vi "add set temp(SubVI).vi"(10 "字符串":string) -> (0 "布尔 3":bool, 2 "连接的字符串":string)   [LabVIEW 2019, in "SubVI.lvlib"]
uses:
  SubVI.lvlib
panel:
  in  "Mode":i32(ring) items=["FastSettle", "NoOvershoot"]
  in  "cancel":bool
  in  "ok":bool
  in  "Rate(K/min)":dbl=10.0 min=0.0 max=10.0
  in  "Temperature(K)":dbl=2.0 min=2.0 max=400.0
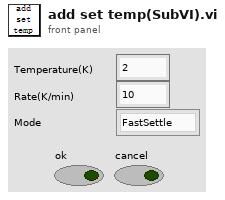
[diagram p1: front panel]
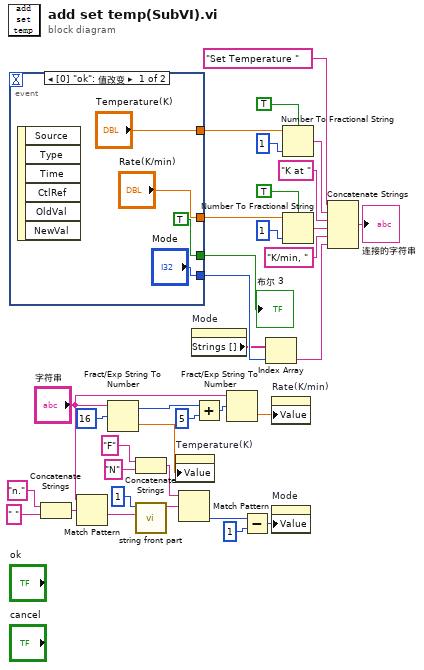
[diagram p0: block diagram]
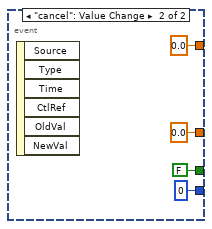
[diagram p2: hidden frame]
diagram:
  n1 = event shown="[0] \"ok\": 值改变" {
    selector: _ -> [_ _]
    dyn-events: _ -> [_ _]
    timeout: _ -> [_ _]
    tunnel: ["Rate(K/min)" 0.0 ("Rate输入")] -> w26
    tunnel: ["Temperature(K)" 0.0 ("Field")] -> w33
    tunnel: [TRUE FALSE] -> w35
    tunnel: ["Mode" 0 ("Approach输入")] -> w23
    event "ok": Value Change {
      n2 = event-data() -> ()  [unwired: 1 in, 6 out]
    }
    event "cancel": Value Change {
      n3 = event-data() -> ()  [unwired: 1 in, 6 out]
    }
  }
  "布尔 3" <- w35
  n4 = Concatenate Strings("n." ("正则表达式"), " " ("字符串")) -> (w5:string)
  n5 = Match Pattern(string="字符串", regular expression=w5) -> (after substring=w8:string)  [unwired: 1 in, 3 out]
  n6 = Fract/Exp String To Number(string="字符串", offset=16 ("偏移量")) -> (offset past number=w18:i32, number=w3:dbl)  [unwired: 2 in]
  n7 = Concatenate Strings("F" ("字符串"), "N" ("字符串")) -> (w11:string)
  n8 = call "string front part.vi"("字符串"=w8, "偏移量(0)"=1) -> ("result string"=w14:string)  [unwired: 9 in]
  n9 = property on="Temperature(K)" class="DigNum (严格)"("Value"=w3) -> ()  [unwired: 2 in, 2 out]
  n10 = Match Pattern(string=w11, regular expression=w14) -> (offset past match=w10:i32)  [unwired: 1 in, 3 out]
  n11 = property on="Mode" class="Ring (严格)"() -> ("Strings []"=w20:string[])  [unwired: 2 in, 2 out]
  n12 = Add(x=w18, y=5) -> (x+y=w17:i32)
  n13 = Fract/Exp String To Number(string="字符串", offset=w17) -> (number=w2:dbl)  [unwired: 2 in, 1 out]
  n14 = Subtract(x=w10, y=1) -> (x-y=w1:i32)
  n15 = Index Array(array=w20, index=w23) -> (element=w22:string)
  n16 = property on="Rate(K/min)" class="DigNum (严格)"("Value"=w2) -> ()  [unwired: 2 in, 2 out]
  n17 = property on="Mode" class="Ring (严格)"("Value"=w1) -> ()  [unwired: 2 in, 2 out]
  n18 = Number To Fractional String(use system decimal point (T)=TRUE ("使用系统小数点(T)"), number=w33, precision (6)=i16 1 ("精度(6)")) -> (F-format string=w31:string)  [unwired: 1 in]
  n19 = Number To Fractional String(use system decimal point (T)=TRUE ("使用系统小数点(T)"), number=w26, precision (6)=i16 1 ("精度(6)")) -> (F-format string=w25:string)  [unwired: 1 in]
  n20 = Concatenate Strings("Set Temperature " ("字符串"), w31, "K at " ("字符串"), w25, "K/min, " ("字符串"), w22) -> (→"连接的字符串":string)
